vi "Drive Motor Test.vi"(0 "On?":bool, 1 "Encoder Refnum":string="Drive Encoder FL", 5 "Drive Back?":bool, 7 "Reset Encoders":bool, 9 "Speed":dbl, 11 "Target Encoder":i32, 12 "Motor Refnum":string="Drive FL") -> (3 "Current Encoder":i32)   [LabVIEW 2014]
uses:
  <vilib>/addons/control/pid/pid.llb/PID (DBL).vi
  <vilib>/addons/control/pid/NI_PID_pid.lvlib
panel:
  in  "PID gains":T1={"proportional gain (Kc)"=1.0, "integral time (Ti, min)"=0.01, "derivative time (Td, min)"=0.0} {"derivative time (Td, min)" format="%.3f"; "integral time (Ti, min)" format="%.3f"; "proportional gain (Kc)" format="%.3f"}
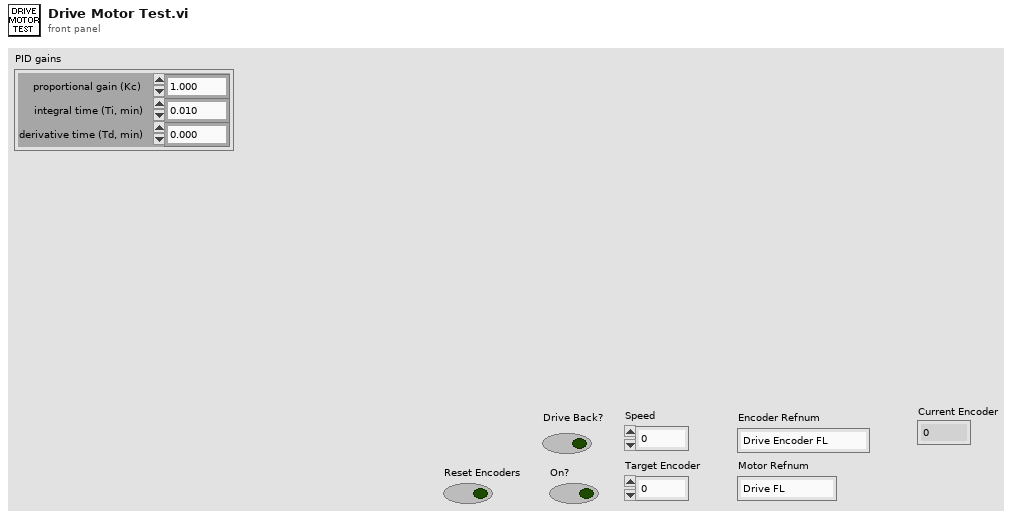
[diagram p1: front panel]
types:
  T1 = cluster{"proportional gain (Kc)":dbl, "integral time (Ti, min)":dbl, "derivative time (Td, min)":dbl}
  T2 = typedef "WPI_CounterDevRef.ctl" = cluster{"DevStatus":errorcluster, "CntIndex":T3}
  T3 = typedef "FPGA_CounterCtrSystemIndex.ctl" = enum8{"Ctr 0", "Ctr 1", "Ctr 2", "Ctr 3", "Ctr 4", "Ctr 5", "Ctr 6", "Ctr 7", "Invalid"}
  T4 = typedef "WPI_MotorControlDeviceRef.ctl" = cluster{"DeviceStatus":errorcluster, "Type":T5, "PWM":cluster{"Controller":T6, "PWM Channel":T7, "DeadBand":T8}, "CAN":cluster{"Device Number":u8, "Control Mode":T9, "Semaphore":T10, "Max Vout":dbl, "TalonSRX Control Mode":T11}, "Invert":bool, "TransformRef":T12, "InvTransformRef":T12}
  T5 = typedef "WPI_MotorControlType.ctl" = enum16{"PWM", "CAN", "CANTalonSRX"}
  T6 = typedef "FPGA_TypedefDigitalModule.ctl" = enum16{"Controller 1"}
  T7 = typedef "FPGA_DIOPWMChannel.ctl" = enum8{"PWM 0", "PWM 1", "PWM 2", "PWM 3", "PWM 4", "PWM 5", "PWM 6", "PWM 7", "PWM 8", "PWM 9", "PWM MXP 0", "PWM MXP 1", "PWM MXP 2", "PWM MXP 3", "PWM MXP 4", "PWM MXP 5", "PWM MXP 6", "PWM MXP 7", "PWM MXP 8", "PWM MXP 9", "Invalid"}
  T8 = typedef "WPI_PWMDeadband.ctl" = cluster{"Name":string, "maxPositivePwm":i32, "minPositivePwm":i32, "centerPwm":i32, "maxNegativePwm":i32, "minNegativePwm":i32, "angularRange":u16}
  T9 = typedef "WPI_CANJaguar_ControlMode.ctl" = enum8{"Percent VBus", "Current", "Speed", "Position", "Voltage"}
  T10 = typedef "Semaphore RefNum" = refnum<k1>
  T11 = typedef "WPI_CANTalonSRX_APIControlMode.ctl" = enum8{"Percent VBus", "Speed", "Position", "Slave", "Unchanged / Invalid"}
  T12 = typedef "WPI_PWMTransform_ConPane.ctl" = refnum<vi>
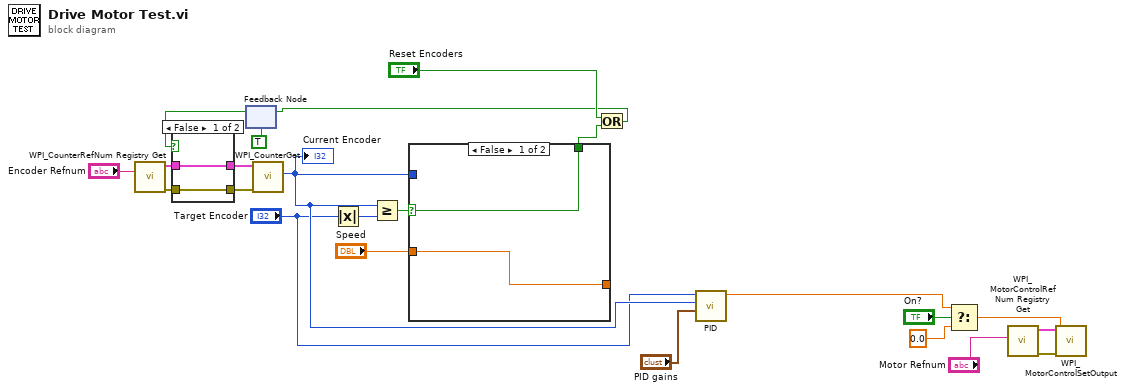
[diagram p0: block diagram]
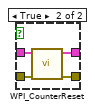
[diagram p2: hidden frame]
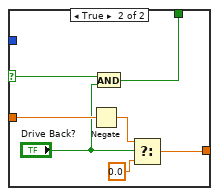
[diagram p3: hidden frame]
diagram:
  n1 = call <vilib>:"WPI_CounterRefNum Registry Get.vi"("refnum name"="Encoder Refnum") -> ("error out"=w15:errorcluster, "CounterDevRef"=w16:T2)  [unwired: 9 in]
  n2 = feedback #1(TRUE ("Reset Tachs")) -> (w20:bool)
  n3 = case shown="False" w20 {
    tunnel: [w25 w27] -> w18
    tunnel: w16 -> [w25 w26]
    tunnel: [w24 w28] -> w19
    tunnel: w15 -> [w24 w29]
    frame False {
    }
    frame True {
      n4 = call <vilib>:"WPI_CounterReset.vi"("error in (no error)"=w29, "CounterDevRef in"=w26) -> ("error out"=w28:errorcluster, "CounterDevRef out"=w27:T2)  [unwired: 8 in]
    }
  }
  n5 = call <vilib>:"WPI_CounterGet.vi"("error in (no error)"=w19, "CounterDevRef in"=w18) -> ("Value"=w4:i32)  [unwired: 4 in, 5 out]
  "Current Encoder" <- w4
  n6 = Absolute Value(x="Target Encoder") -> (abs(x)=w23:i32)
  n7 = Greater Or Equal?(x=w4, y=w23) -> (x >= y?=w14:bool)
  n8 = case shown="False" w14 {
    selector: w14 -> [w30 w33]
    tunnel: w4 -> [_ _]
    tunnel: "Speed" -> [w31 w37]
    tunnel: [w31 w35] -> _
    tunnel: [w30 w32] -> w7
    frame False {
    }
    frame True {
      n9 = Negate(x=w37) -> (-x=w38:dbl)
      n10 = And(x=w33, y="Drive Back?") -> (x .and. y?=w32:bool)
      n11 = Select(t=w38, s="Drive Back?", f=0.0) -> (s? t:f=w35:dbl)
    }
  }
  n12 = Or(x="Reset Encoders", y=w7) -> (x .or. y?=w5:bool)
  n13 = feedback-in #1(w5) -> ()
  n14 = call-poly <vilib>:"PID.vi"("PID gains"="PID gains", "process variable"=w4, "setpoint"="Target Encoder") -> ("output"=w1:dbl)  [unwired: 7 in, 1 out]
  n15 = Select(t=w1, s="On?", f=0.0) -> (s? t:f=w9:dbl)
  n16 = call <vilib>:"WPI_MotorControlRefNum Registry Get.vi"("refnum name"="Motor Refnum") -> ("error out"=w11:errorcluster, "MotorControlDevRef"=w10:T4)  [unwired: 9 in]
  n17 = call <vilib>:"WPI_MotorControlSetOutput.vi"("error in (no error)"=w11, "Output"=w9, "MotorControlDevRef"=w10) -> ()  [unwired: 6 in, 3 out]
